vi "Add Sample (ref).vi"(0 "Session Handle in":T1, 5 "Sample Name":string, 7 "Value":dbl, 9 "Timestamp":timestamp format="%<%x %.3X>T", 11 "error in (no error)":errorcluster, 12 "Labels":map{string, string}(c390)) -> (4 "Session Handle out":T1, 15 "error out":errorcluster)   [LabVIEW 2020, in "Metric Session.lvclass"]
uses:
  Metric Session.lvclass
  Typedefs/Session Handle.ctl
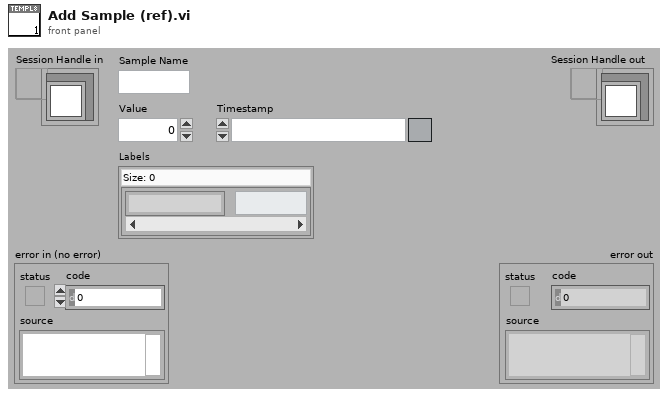
[diagram p1: front panel]
types:
  T1 = typedef "Metric Session.lvclass/Session Handle.ctl" = refnum<data-value>
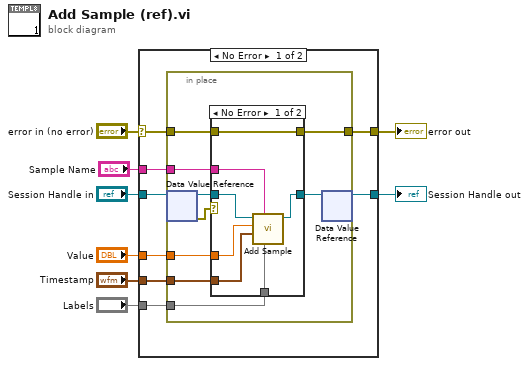
[diagram p0: block diagram]
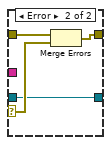
[diagram p2: hidden frame]
diagram:
  n1 = case shown="No Error" "error in (no error)" {
    selector: "error in (no error)" -> [w14 w37]
    tunnel: "Session Handle in" -> [w16 w38]
    tunnel: [w15 w38] -> w7
    tunnel: [w13 w37] -> w6
    tunnel: "Sample Name" -> [w12 _]
    tunnel: "Value" -> [w11 _]
    tunnel: "Timestamp" -> [w10 _]
    tunnel: "Labels" -> [w9 _]
    frame No Error {
      n2 = in-place {
        in-place-border: w14 -> [w21]
        in-place-border: [w24] -> w13
        in-place-border: w12 -> [w20]
        in-place-border: w11 -> [w19]
        in-place-border: w10 -> [w18]
        in-place-border: w9 -> [w17]
        n3 = in-place-dvr #1(w16) -> (w25:refnum<class "Metric Session.lvclass">, w22:errorcluster)
        n4 = case shown="No Error" w22 {
          selector: w22 -> [_ w35]
          tunnel: w25 -> [w31 w33]
          tunnel: [w32 w34] -> w24
          tunnel: [w30 w33] -> w23
          tunnel: w21 -> [w32 w36]
          tunnel: w20 -> [w29 _]
          tunnel: w19 -> [w28 _]
          tunnel: w18 -> [w27 _]
          tunnel: w17 -> [w26 _]
          frame No Error {
            n5 = call-dynamic "Add Sample.vi"("Labels"=w26, "Sample Name"=w29, "Timestamp"=w27, "Value"=w28, "Metric in"=w31) -> ("Metric out"=w30:refnum<class "Metric Session.lvclass">)  [unwired: 5 in, 1 out]
          }
          frame Error {
            n6 = Merge Errors(w36, w35) -> (w34:errorcluster)
          }
        }
        n7 = in-place-dvr #1(w23) -> (w15:T1)  [unwired: 1 out]
      }
    }
    frame Error {
    }
  }
  "Session Handle out" <- w7
  "error out" <- w6
